vi "Write configuration.vi"(8 "error in":errorcluster, 10 "folder configuration":refnum<class "CEF_serializable node folder configuration.lvclass">, 11 "CEF_serializable node folder in":refnum<class "CEF_serializable node folder.lvclass">) -> (0 "error out":errorcluster, 3 "CEF_serializable node folder out":refnum<class "CEF_serializable node folder.lvclass">)   [LabVIEW 2023, in "CEF_serializable node folder.lvclass"]
doc: "Copyright 2017 National Instruments Corporation\n\nLicensed under the Apache License, Version 2.0 (the \"License\"); you may not use this file except in compliance with the License. You may obtain a copy of the License at http://www.apache.org/licenses/LICENSE-2.0\nUnless required by applicable law or agreed to in writing, software distributed under the License is distributed on an \"AS IS\" BASIS, WITHOUT WARRANTIES OR CONDITIONS OF ANY KIND, either express or implied. See the License for the specific language governing permissions and limitations under the License."
uses:
  CEF_serializable node folder.lvclass
  CEF_serializable node folder.lvclass/CEF_serializable node folder.ctl
  folder configuration/CEF_serializable node folder configuration.lvclass
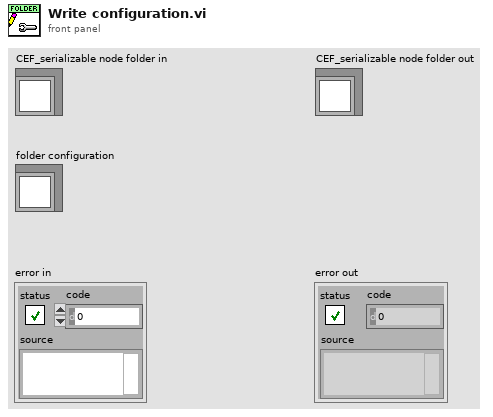
[diagram p1: front panel]
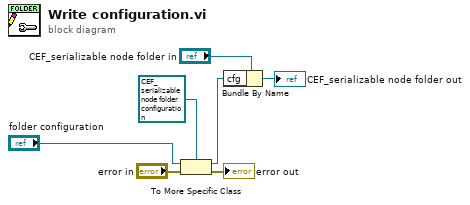
[diagram p0: block diagram]
diagram:
  n1 = To More Specific Class(target class=refnum<class "CEF_serializable node folder configuration.lvclass"> refnum ("folder configuration"), reference="folder configuration", error in="error in") -> (specific class reference=w2:refnum<class "CEF_serializable node folder configuration.lvclass">, error out=→"error out":errorcluster)
  n2 = Bundle By Name(cluster="CEF_serializable node folder in", "cfg"=w2) -> (→"CEF_serializable node folder out":refnum<class "CEF_serializable node folder.lvclass">)
